vi "PROJE ÖDEVİ.vi"() -> ()   [LabVIEW 2018]
uses:
  <vilib>/MakerHub/LINX/Public/Peripherals/Analog/Analog Read 1 Chan.vi
  <vilib>/MakerHub/LINX/Public/Peripherals/Analog/Analog Read N Chans.vi
  <vilib>/MakerHub/LINX/Private/Local IO/LinxAnalogRead.vi
  <vilib>/MakerHub/LINX/Public/Utilities/Check Channel.vi
  <vilib>/MakerHub/LINX/Public/Utilities/Open Serial.vi
  <vilib>/MakerHub/LINX/Private/Utilties/Generate Error.vi
  <vilib>/MakerHub/LINX/LMH-LINX.lvlib
panel:
  out "Sıcak Mod":bool
  out "Fan Modu":bool
  out "Soğuk Mod":bool
  out "Sıcaklık Grafiği":dbl(graph)
  out "Termometre":dbl(slide) scale=0.0..100.0
  out "Sıcaklık Değeri":dbl
  # "OTOMOTİK  KLİMA SİSTEMİ"
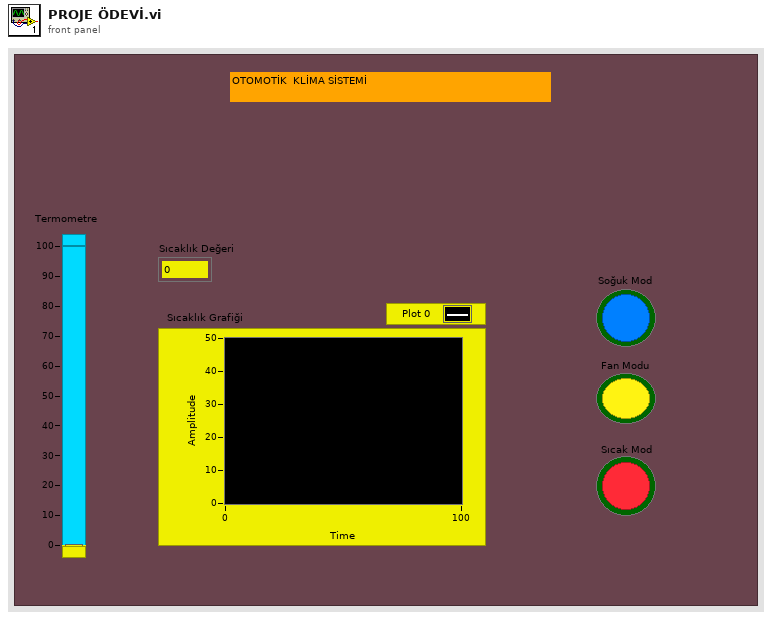
[diagram p1: front panel]
types:
  T1 = typedef "LMH-LINX.lvlib/LINX Ref.ctl" = cluster{"IO":T2, "Interface":T3, "LINX Device Config":T4}
  T2 = typedef "LMH-LINX.lvlib/Platform.ctl" = enum16{"Remote", "Local"}
  T3 = typedef "LMH-LINX.lvlib/Interface.ctl" = enum16{"Serial", "TCP"}
  T4 = typedef "LMH-LINX.lvlib/Device.lvlib/LINX Device Config.ctl" = cluster{"Interface":T3, "COM Port":refnum<visa-resource-name>, "TCP Configuration":T5, "Device Family":u8, "Device ID":u8, "Device Name":string, "TCP Ref":refnum<k5>, "Channels":T6}
  T5 = typedef "LMH-LINX.lvlib/Device.lvlib/TCP Config.ctl" = cluster{"IP Address":string, "Port":u16}
  T6 = typedef "LMH-LINX.lvlib/Channels.ctl" = cluster{"DI":u8[], "DO":u8[], "AI":u8[], "AO":u8[], "PWM":u8[], "QE":u8[], "UART":u8[], "I2C 2":u8[], "SPI":u8[], "CAN":u8[], "Servo":u8[], "AI Ref (V)":dbl, "AI Resolution (Bits)":u8, "AO Ref (V)":dbl, "AO Resolution (Bits)":u8}
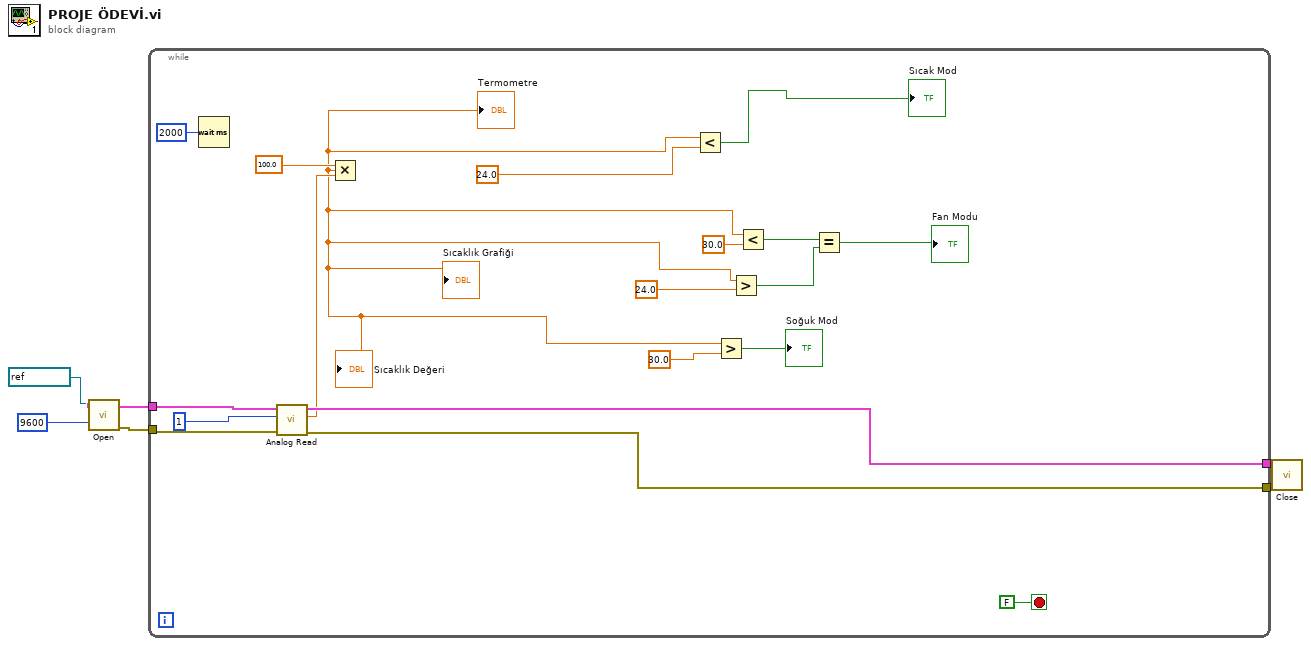
[diagram p0: block diagram]
diagram:
  n1 = call-poly <vilib>:"Open.vi"("Baud Rate Override"=u32 9600, "Serial Port"=refnum<visa-resource-name> "COM3") -> ("Error Out"=w4:errorcluster, "LINX Resource"=w6:T1)  [unwired: 7 in, 1 out]
  n2 = while {
    tunnel: w6 -> [w25]
    tunnel: [w24] -> w5
    tunnel: w4 -> [w23]
    tunnel: [w22] -> w3
    stop <- FALSE stop-if-true
    n3 = Wait (ms)(milliseconds to wait=u32 2000) -> ()  [unwired: 1 out]
    n4 = call-poly <vilib>:"Analog Read.vi"("Error In"=w23, "Analog Channel"=u8 1, "LINX Resource"=w25) -> ("Error Out"=w22:errorcluster, "Voltage"=w21:dbl, "LINX Resource"=w24:T1)  [unwired: 5 in, 1 out]
    n5 = Multiply(x=100.0, y=w21) -> (x*y=w10:dbl)
    "Sıcaklık Değeri" <- w10
    "Termometre" <- w10
    "Sıcaklık Grafiği" <- w10
    n6 = Less?(x=w10, y=24.0) -> (x < y?=→"Sıcak Mod":bool)
    n7 = Greater?(x=w10, y=30.0) -> (0:→"Soğuk Mod":bool)
    n8 = Greater?(x=w10, y=24.0) -> (0:w8:bool)
    n9 = Less?(x=w10, y=30.0) -> (x < y?=w7:bool)
    n10 = Equal?(x=w7, y=w8) -> (x = y?=→"Fan Modu":bool)
  }
  n11 = call <vilib>:"Close.vi"("Error In"=w3, "LINX Resource"=w5) -> ()  [unwired: 9 in, 1 out]
